vi "midiOutShortMsg.vi"(8 "error in":errorcluster, 10 "data":u32, 11 "midi in":refnum<class "midi.lvclass">) -> (0 "error out":errorcluster, 3 "midi out":refnum<class "midi.lvclass">)   [LabVIEW 2020, in "midi.lvclass"]
doc: "The midiOutShortMsg function sends a short MIDI message to the specified MIDI output device.\n\nMIDI message. The message is packed into a DWORD value with the first byte of the message in the low-order byte. The message is packed into this parameter as follows:\nWord High -> High Order -> Not Used\nWord High -> Low Order -> The second byte of MIDI data (when needed)\nWord Low -> High Order -> The first byte of MIDI data (when needed).\nWord Low -> Low Order -> The MIDI status.\n\nThe two MIDI data bytes are optional, depending on the MIDI status byte. When a series of messages have the same status byte, the status byte can be omitted from messages after the first one in the series, creating a running status. Pack a message for running status as follows:\nWord High -> High Order -> Not used.\nWord High -> Low Order -> Not used.\nWord Low -> High Order -> The second byte of MIDI data (when needed).\nWord Low -> Low Order -> The first byte of MIDI data."
uses:
  midi.lvclass
  midi.lvclass/midi.ctl
  winmm.dll
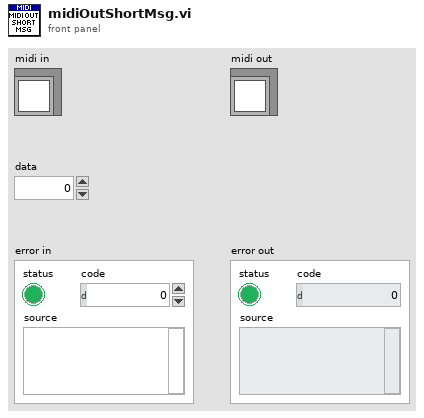
[diagram p1: front panel]
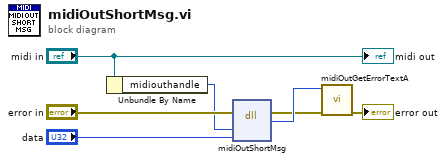
[diagram p0: block diagram]
diagram:
  n1 = Unbundle By Name("midi in") -> ("midiouthandle"=w3:u64)
  n2 = dll-call lib="winmm.dll" fn="midiOutShortMsg"(error in="error in", "hmo"=w3, "dwMsg"="data") -> (error out=w5:errorcluster, "error code"=w6:i32)  [unwired: 4 in, 1 out]
  n3 = call "midiOutGetErrorTextA.vi"("error in"=w5, "Error Code"=w6) -> ("error out"=→"error out":errorcluster)  [unwired: 9 in]
  "midi out" <- "midi in"
